vi "Volatus Meta Value Lookup.vi"(6 "Exact Value (F)":bool, 7 "Don't Recurse Past Match (F)":bool, 8 "error in (no error)":errorcluster, 9 "Value":string, 10 "Meta Name":T1, 11 "Config Lookup (New)":refnum<class "Config Lookup.lvclass">) -> (0 "error out":errorcluster, 3 "Config Lookup out":refnum<class "Config Lookup.lvclass">)   [LabVIEW 2020, in "VolatusConfig.lvlib"]
uses:
  VolatusConfig.lvlib
  lv-cdm/CDM-Config/Config Filter/Config Lookup.lvclass
  Meta Name.ctl
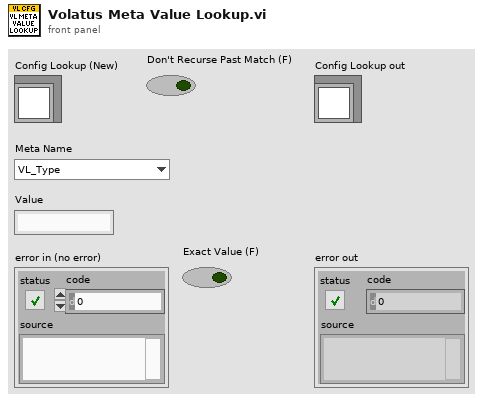
[diagram p1: front panel]
types:
  T1 = typedef "VolatusConfig.lvlib/Meta Name.ctl" = enum16{"VL_Type", "VL_Node_IP", "VL_Node_Type", "VL_Task_Type", "VL_Group_Type", "VL_Channel_Type", "VL_Channel_DataType", "VL_Config_Version", "VL_Overlay_Type"}
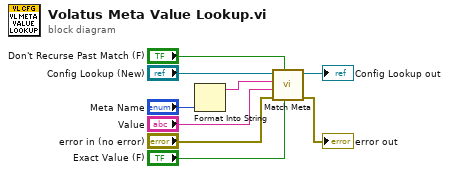
[diagram p0: block diagram]
diagram:
  n1 = Format Into String("Meta Name") -> (resulting string=w8:string)  [unwired: 3 in, 1 out]
  n2 = call "Match Meta.vi"("Exact Value (F)"="Exact Value (F)", "Don't Recurse Past Match (F)"="Don't Recurse Past Match (F)", "error in (no error)"="error in (no error)", "Value (Any)"="Value", "Name"=w8, "Config Lookup (New)"="Config Lookup (New)") -> ("error out"=→"error out":errorcluster, "Config Lookup out"=→"Config Lookup out":refnum<class "Config Lookup.lvclass">)  [unwired: 4 in]
